vi "PXF4_get_PV_MV.vi"(8 "error in":errorcluster, 11 "Modbus Master in":refnum<class "Modbus Master.lvclass">) -> (0 "error out":errorcluster, 1 "SV":dbl format="%.1f", 2 "PV":dbl format="%.1f", 3 "Modbus Master out":refnum<class "Modbus Master.lvclass">, 4 "Output":bool)   [LabVIEW 2019]
uses:
  <vilib>/NI/Modbus Library/API/Master/Modbus Master.lvclass
panel:
  out "MV1":u16
  out "SV_raw":u16
  out "PV_raw":u16
  out "register values":u16[](array[numeric])
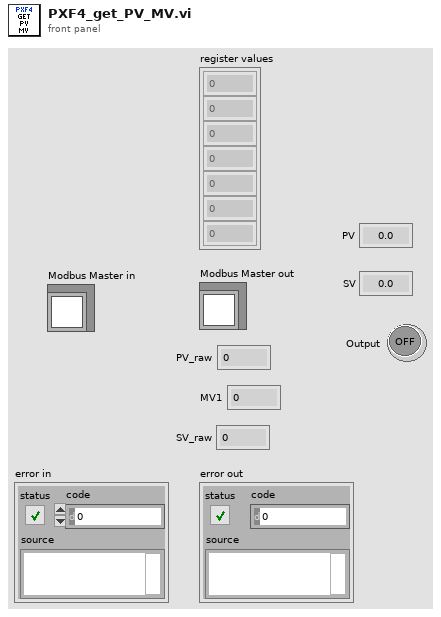
[diagram p1: front panel]
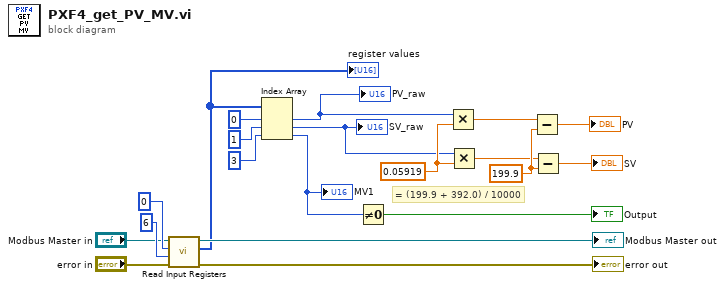
[diagram p0: block diagram]
diagram:
  w5 = 199.9 ("y")
  w8 = 0.05919 ("y")
  # "= (199.9 + 392.0) / 10000"
  n1 = call-dynamic "Read Input Registers.vi"("error in"="error in", "number of inputs"=u16 6, "starting address"=u16 0, "Modbus master in"="Modbus Master in") -> ("error out"=→"error out":errorcluster, "register values"=w15:u16[], "Modbus master out"=→"Modbus Master out":refnum<class "Modbus Master.lvclass">)  [unwired: 5 in]
  "register values" <- w15
  n2 = Index Array(array=w15, index #1=0 ("index"), index #2=1 ("index"), index #3=3 ("index")) -> (element #1=w6:u16, element #2=w7:u16, element #3=w10:u16)
  "PV_raw" <- w6
  "SV_raw" <- w7
  "MV1" <- w10
  n3 = Not Equal To 0?(x=w10) -> (x != 0?=→"Output":bool)
  n4 = Multiply(x=w6, y=w8) -> (x*y=w4:dbl)
  n5 = Multiply(x=w7, y=w8) -> (x*y=w3:dbl)
  n6 = Subtract(x=w4, y=w5) -> (x-y=→"PV":dbl)
  n7 = Subtract(x=w3, y=w5) -> (x-y=→"SV":dbl)
